vi "list_all_switch_states.vi"(10 "instrument name":string, 11 "PrepLine\nobjects":refnum<class "PrepLineObject.lvclass">[](array[class])) -> ()   [LabVIEW 2013]
doc: "goes through all PrepLineOnject Switches that belong to \"instrument name\" and lists their states in an array"
uses:
  PrepLineObject.lvclass
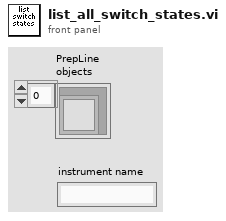
[diagram p1: front panel]
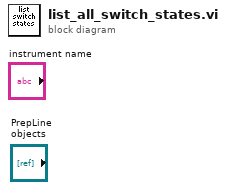
[diagram p0: block diagram]
diagram:
